vi "while_v0_v14.vi"() -> ()   [LabVIEW 2009]
panel:
  in  "Bottom":u16(slide)=182 scale=300.0..0.0
  in  "Right":u16(slide)=335 scale=0.0..400.0
  in  "Top":u16(slide)=71 scale=300.0..0.0
  in  "Culoare":u32(colorbox)=16716337
  in  "Left":u16(slide)=79 scale=0.0..400.0
  in  "stop":bool
  out "Picture":picture
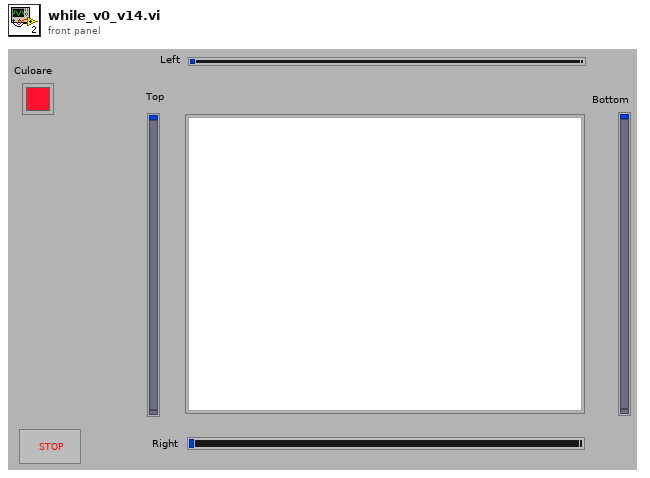
[diagram p1: front panel]
types:
  T1 = cluster{"Left":u16, "Top":u16, "Right":u16, "Bottom":u16}
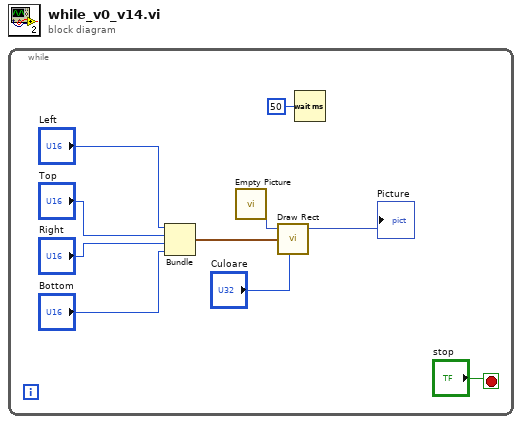
[diagram p0: block diagram]
diagram:
  n1 = while {
    stop <- "stop" stop-if-true
    n2 = Bundle("Left"="Left", "Top"="Top", "Right"="Right", "Bottom"="Bottom") -> (w9:T1)  [unwired: 1 in]
    n3 = call "Empty Picture"() -> ("empty picture"=w1:picture)
    n4 = call <vilib>:"Draw Rect.vi"("picture"=w1, "rect"=w9, "color(black)"="Culoare") -> ("new picture"=→"Picture":picture)  [unwired: 6 in]
    n5 = Wait (ms)(milliseconds to wait=u32 50) -> ()  [unwired: 1 out]
  }
